vi "niDTS BT Tx Test Example.vi"() -> ()   [LabVIEW 2014]
uses:
  Tx Test/Includes/niDTS BT Tx Test INC IBE Results.ctl
  Tx Test/Includes/niDTS BT Tx Test INC Character Results.ctl
  Tx Test/Includes/niDTS BT Tx Test INC CFO Resutls.ctl
  Tx Test/Includes/niDTS BT Tx Test INC TXP Results.ctl
  Tx Test/Includes/niDTS BT Tx Test INC OBW Results.ctl
  BDR Tx Test/Includes/niDTS BT BDR Tx Test INC Results.ctl
  CommLib/Includes/niDTS Comm INC CLI Login.ctl
  EDR Tx Test/Includes/niDTS BT EDR Tx Test INC Results.ctl
  Tx Test/Includes/niDTS BT Tx Test INC DEVM Results.ctl
  Tx Test/Includes/niDTS BT Tx Test INC CF Stability Results.ctl
  LE Tx Test/Includes/niDTS BT LE Tx Test INC Results.ctl
  LE Tx Test/Includes/niDTS BT LE Tx Test INC Parameters.ctl
  Tx Test/Includes/niDTS BT Tx Test INC BD Payload Data.ctl
  Tx Test/Includes/niDTS BT Tx Test INC Modulation Characteristics.ctl
  Includes/niDTS BT INC TXP Measurement Parameters.ctl
  LE Tx Test/Includes/niDTS BT INC LE IBE Measurement Parameters.ctl
  Includes/niDTS BT DUT INC Trigger.ctl
  EDR Tx Test/Includes/niDTS BT EDR Tx Test INC Parameters.ctl
  EDR Tx Test/Includes/niDTS BT INC EDR Packet Type.ctl
  EDR Tx Test/Includes/niDTS BT INC EDR Data Rate.ctl
  EDR Tx Test/Includes/niDTS BT INC EDR Burst Sync.ctl
  EDR Tx Test/Includes/niDTS BT INC EDR ModAcc Measurement Parameters.ctl
  EDR Tx Test/Includes/niDTS BT INC EDR IBE Measurement Parameters.ctl
  BDR Tx Test/Includes/niDTS BT BDR Tx Test INC Parameters.ctl
  BDR Tx Test/Includes/niDTS BT INC BDR Packet Type.ctl
  Includes/niDTS BT INC OBW Measurement Parameters.ctl
  BDR Tx Test/Includes/niDTS BT INC BDR ACP Measurement Parameters.ctl
  Framework/Logger/Includes/niDTS Logger INC File Parameters.ctl
  TestStand/Station/Objects/SystemDutHandle/niDTS SystemDutHandle.lvclass
  Framework/niDTS Framework.lvlib
  niDTS BT.lvlib
  TestStand/niDTS TestStand.lvlib
  Plugins/niBCM4350 BT/niBCM4350 BT.lvlib
  Plugins/niLEDTM BT/niLEDTM BT.lvlib
  Plugins/niWTM Loopback/niWTM Loopback.lvlib
  Framework/Logger/Listener/Viewer/niDTS Logger Listener Viewer.lvclass
  CommLib/niDTS CommLib.lvlib
panel:
  in  "Keep Log Open":bool
  in  "ResultsIndex":u8=1
  in  "Tab Control":enum32{"BDR", "EDR", "LE TP"}(tab)
  out "BDR Results":T6={"ACP Results"={"Measurement Status"=TRUE, "Reference Channel Power (dBm)"=-9.745, "Upper Channel Power (dBm)"=-37.144, "Lower Channel Power (dBm)"=-37.251, "Total Channel Powers (dBm)"=[-83.632, -78.931, -37.144, -9.745, -37.251, -79.301, -83.479]}, "DF1/DF2"={"Average df1Avg (Hz)"=161011.015625, "Max df1Max (Hz)"=161733.942382812, "Min df1Max (Hz)"=160248.126464844, "Measurement Status df1"=TRUE, "Average  df2Avg/Average df1Avg"=nan, "Average df2Avg (Hz)"=nan, "Max df2Max (Hz)"=nan, "Min df2Max (Hz)"=nan, "Measurement Status df2"=FALSE}, "CFO"={"Max ICFT (Hz)"=548.11181640625, "Max Carrier Drift (Hz)"=-686.029418945312, "Max Carrier Drift/50us (Hz)"=173.238983154297, "LE MaxPayloadBlockFreqOffset (Hz)"=nan, "LE MaxCarrierDrift/55us (Hz)"=nan}, "TXP Resutls"={"Average Burst Power (dBm)"=-9.843, "Peak Burst Power (dBm)"=-9.8, "EdrRelativePower (dB)"=-0.01}, "OBW Resutls"={"OBW (Hz)"=908872.719017752, "Start Frequency (Hz)"=-438547.728652488, "Stop Frequency (Hz)"=470324.990365264}} {"OBW Resutls"."Stop Frequency (Hz)" format="%#_4p"; "OBW Resutls"."Start Frequency (Hz)" format="%#_4p"}
  out "USL":T7={"ACP Results"={"Measurement Status"=FALSE, "Reference Channel Power (dBm)"=23.0, "Upper Channel Power (dBm)"=-20.0, "Lower Channel Power (dBm)"=-20.0, "Total Channel Powers (dBm)"=[]}, "DF1/DF2"={"Average df1Avg (Hz)"=175000.0, "Max df1Max (Hz)"=inf, "Min df1Max (Hz)"=inf, "Measurement Status df1"=FALSE, "Average  df2Avg/Average df1Avg"=inf, "Average df2Avg (Hz)"=175000.0, "Max df2Max (Hz)"=inf, "Min df2Max (Hz)"=inf, "Measurement Status df2"=FALSE}, "CFO"={"Max ICFT (Hz)"=75000.0, "Max Carrier Drift (Hz)"=40000.0, "Max Carrier Drift/50us (Hz)"=20000.0, "LE MaxPayloadBlockFreqOffset (Hz)"=nan, "LE MaxCarrierDrift/55us (Hz)"=nan}, "TXP Resutls"={"Average Burst Power (dBm)"=20.0, "Peak Burst Power (dBm)"=23.0, "EdrRelativePower (dB)"=inf}, "OBW Resutls"={"OBW (Hz)"=1500000.0, "Start Frequency (Hz)"=0.0, "Stop Frequency (Hz)"=750000.0}} {"OBW Resutls"."Stop Frequency (Hz)" format="%#_4p"; "OBW Resutls"."Start Frequency (Hz)" format="%#_4p"}
  out "LSL":T7={"ACP Results"={"Measurement Status"=FALSE, "Reference Channel Power (dBm)"=-inf, "Upper Channel Power (dBm)"=-inf, "Lower Channel Power (dBm)"=-inf, "Total Channel Powers (dBm)"=[]}, "DF1/DF2"={"Average df1Avg (Hz)"=140000.0, "Max df1Max (Hz)"=-inf, "Min df1Max (Hz)"=-inf, "Measurement Status df1"=FALSE, "Average  df2Avg/Average df1Avg"=-inf, "Average df2Avg (Hz)"=-inf, "Max df2Max (Hz)"=115000.0, "Min df2Max (Hz)"=0.0, "Measurement Status df2"=FALSE}, "CFO"={"Max ICFT (Hz)"=-75000.0, "Max Carrier Drift (Hz)"=-40000.0, "Max Carrier Drift/50us (Hz)"=-20000.0, "LE MaxPayloadBlockFreqOffset (Hz)"=nan, "LE MaxCarrierDrift/55us (Hz)"=nan}, "TXP Resutls"={"Average Burst Power (dBm)"=-inf, "Peak Burst Power (dBm)"=-inf, "EdrRelativePower (dB)"=-inf}, "OBW Resutls"={"OBW (Hz)"=0.0, "Start Frequency (Hz)"=-750000.0, "Stop Frequency (Hz)"=0.0}} {"OBW Resutls"."Stop Frequency (Hz)" format="%#_4p"; "OBW Resutls"."Start Frequency (Hz)" format="%#_4p"}
  out "x > y?":T8={"ACP Results"={"Measurement Status"=TRUE, "Reference Channel Power dBm"=TRUE, "Upper Channel Power dBm"=TRUE, "Lower Channel Power dBm"=TRUE, "Total Channel Powers dBm"=[]}, "DF1/DF2"={"Average df1Avg"=TRUE, "Max df1Max"=TRUE, "Min df1Max"=TRUE, "Measurement Status df1"=TRUE, "Average  df2Avg/Average df1Avg"=FALSE, "Average df2Avg"=FALSE, "Max df2Max"=FALSE, "Min df2Max 2"=FALSE, "Measurement Status df2"=FALSE}, "CFO"={"Max ICFT Hz"=TRUE, "Max Carrier Drift Hz"=TRUE, "Max Carrier Drift/50us Hz"=TRUE, "LE Max Block Freq Offset, Hz"=FALSE, "LE Max Carrier Drift/55us Hz"=FALSE}, "TXP Resutls"={"Average Burst Power"=TRUE, "Peak Burst Power"=TRUE, "EdrRelativePower"=TRUE}, "OBW Resutls"={"OBW"=TRUE, "Start Frequency"=TRUE, "Stop Frequency"=TRUE}}
  out "x < y?":T8={"ACP Results"={"Measurement Status"=FALSE, "Reference Channel Power dBm"=TRUE, "Upper Channel Power dBm"=TRUE, "Lower Channel Power dBm"=TRUE, "Total Channel Powers dBm"=[]}, "DF1/DF2"={"Average df1Avg"=TRUE, "Max df1Max"=TRUE, "Min df1Max"=TRUE, "Measurement Status df1"=FALSE, "Average  df2Avg/Average df1Avg"=FALSE, "Average df2Avg"=FALSE, "Max df2Max"=FALSE, "Min df2Max 2"=FALSE, "Measurement Status df2"=FALSE}, "CFO"={"Max ICFT Hz"=TRUE, "Max Carrier Drift Hz"=TRUE, "Max Carrier Drift/50us Hz"=TRUE, "LE Max Block Freq Offset, Hz"=FALSE, "LE Max Carrier Drift/55us Hz"=FALSE}, "TXP Resutls"={"Average Burst Power"=TRUE, "Peak Burst Power"=TRUE, "EdrRelativePower"=TRUE}, "OBW Resutls"={"OBW"=TRUE, "Start Frequency"=TRUE, "Stop Frequency"=TRUE}}
  in  "BDR Tx Input Parameters":T9={"Channel"=0, "Dut Tx Power (dBm)"=-10.0, "Auto Level"=FALSE, "External Attenuation (dB)"=0.0, "BDR Packet type"=enum."DH1", "Payload Data"=enum."AUTO", "Burst Sync"=enum."PREamble", "Packet length (bytes)"=-1, "BD ADDRESS"="\u0000\u0000\u0000\u0000\u0000\u0000000000000000", "Modulation Measurement"={"ModAcc Enable"=TRUE, "CFO Enable"=TRUE, "Character Select"=enum."BOTH", "Averages"=1, "Averaging Mode"=enum."RMS", "Measurement Duration (Symbols)"=-1, "Measurement Offset (Symbols)"=0}, "Trace Enable"=FALSE, "OBW Measurement"={"OBW Enable"=TRUE, "OBW Averages"=1, "Averaging Type"=enum."RMS", "Measurement Interval Mode"=enum."AUTO", "Measurement Interval Length (sec)"=0.005}, "TXP Measurement"={"TXP Power Enable"=TRUE, "TXP Averages"=1, "Averaging Type"=enum."RMS"}, "IBE Measurement"={"IBE Enable"=TRUE, "IBE Averages"=1, "Averaging Type"=enum."RMS", "Numbe of Channels"=7, "Channel Mode"=enum."Centered", "Measurement Interval Mode"=enum."AUTO", "Measurement Interval Length (sec)"=0.005}, "Trigger"={"MinQuietTimeDuration (sec)"=0.0001, "TriggerDelay (sec)"=0.0, "TriggerEdge"=enum."RISing", "TriggerSource"=enum."RF0", "TriggerThreshold (dB)"=-20.0, "TriggerTimeout (sec)"=10.0}} {"Trigger"."MinQuietTimeDuration (sec)" format="%#_6p"}
  out "USL EDR":T17={"IBE Results"={"Measurement Status"=FALSE, "Reference Channel Power (dBm)"=23.0, "Upper Channel Power (dBm)"=-20.0, "Lower Channel Power (dBm)"=-20.0, "Total Channel Powers (dBm)"=[]}, "DEVM"={"Average RMS DEVM (%)"=20.0, "Max Peak DEVM (%)"=35.0, "99% DEVM (%)"=30.0}, "CF Stability"={"Average Inital Freq Error (Hz)"=75000.0, "Max Initial Freq Error (Hz)"=75000.0, "Average Block Abs Freq Error (Hz)"=75000.0, "Max Block Abs Freq Error (Hz)"=75000.0, "Average Block Rel Freq Error (Hz)"=10000.0, "MaxBlockRel Freq Error (Hz)"=10000.0}, "TXP Resutls"={"Average Burst Power (dBm)"=23.0, "Peak Burst Power (dBm)"=20.0, "EdrRelativePower (dB)"=4.0}}
  out "EDR Results":T20
  out "LSL EDR":T17={"IBE Results"={"Measurement Status"=FALSE, "Reference Channel Power (dBm)"=-inf, "Upper Channel Power (dBm)"=-inf, "Lower Channel Power (dBm)"=-inf, "Total Channel Powers (dBm)"=[]}, "DEVM"={"Average RMS DEVM (%)"=0.0, "Max Peak DEVM (%)"=0.0, "99% DEVM (%)"=0.0}, "CF Stability"={"Average Inital Freq Error (Hz)"=-75000.0, "Max Initial Freq Error (Hz)"=-75000.0, "Average Block Abs Freq Error (Hz)"=-75000.0, "Max Block Abs Freq Error (Hz)"=-75000.0, "Average Block Rel Freq Error (Hz)"=-10000.0, "MaxBlockRel Freq Error (Hz)"=-10000.0}, "TXP Resutls"={"Average Burst Power (dBm)"=-inf, "Peak Burst Power (dBm)"=-inf, "EdrRelativePower (dB)"=-1.0}}
  out "EDR":T21
  out "EDR":T21
  in  "EDR Tx Input Parameters":T22={"Channel"=0, "Dut Tx Power  (dBm)"=-10.0, "Auto Level"=FALSE, "External Attenuation (dB)"=0.0, "EDR Packet type"=enum."DH1", "Data Rate"=2, "Payload Data"=enum."PN9", "Burst Sync"=enum."PREamble", "Packet Length, bytes"=-1, "BD ADDRESS"="\u0000\u0000\u0000\u0000\u0000\u0000000000000000", "Trace Enable"=FALSE, "EDR ModAcc Measurement"={"DEVM Enable"=TRUE, "Averages"=1, "Averaging Mode"=enum."RMS", "Measurement Duration (bytes)"=-1, "Measurement Offset (bytes)"=0}, "TXP Measurement"={"TXP Power Enable"=TRUE, "TXP Averages"=1, "Averaging Type"=enum."RMS"}, "IBE  Measurement"={"IBE Enable"=TRUE, "IBE Averages"=1, "Averaging Type"=enum."RMS", "Numbe of Channels"=7, "Channel Mode"=enum."Centered", "Measurement Interval Mode"=enum."AUTO", "Measurement Interval Length (sec)"=0.005}, "Trigger"={"MinQuietTimeDuration (sec)"=0.0001, "TriggerDelay (sec)"=0.0, "TriggerEdge"=enum."RISing", "TriggerSource"=enum."RF0", "TriggerThreshold (dB)"=-20.0, "TriggerTimeout (sec)"=10.0}} {"Trigger"."MinQuietTimeDuration (sec)" format="%#_6p"; "Data Rate" min=2 max=3 step=1}
  out "LE USL":T28={"LE IBE Results"={"Measurement Status"=FALSE, "Reference Channel Power (dBm)"=13.0, "Upper Channel Power (dBm)"=-20.0, "Lower Channel Power (dBm)"=-20.0, "Total Channel Powers (dBm)"=[]}, "DF1/DF2"={"Average df1Avg (Hz)"=nan, "Max df1Max (Hz)"=nan, "Min df1Max (Hz)"=nan, "Measurement Status df1"=FALSE, "Average  df2Avg/Average df1Avg"=inf, "Average df2Avg (Hz)"=nan, "Max df2Max (Hz)"=nan, "Min df2Max (Hz)"=nan, "Measurement Status df2"=FALSE}, "CFO"={"Max ICFT (Hz)"=inf, "Max Carrier Drift (Hz)"=inf, "Max Carrier Drift/50us (Hz)"=inf, "LE MaxPayloadBlockFreqOffset (Hz)"=0.0, "LE MaxCarrierDrift/55us (Hz)"=0.0}, "TXP Resutls"={"Average Burst Power (dBm)"=23.0, "Peak Burst Power (dBm)"=20.0, "EdrRelativePower (dB)"=inf}}
  out "LE LSL":T28={"LE IBE Results"={"Measurement Status"=FALSE, "Reference Channel Power (dBm)"=-inf, "Upper Channel Power (dBm)"=-inf, "Lower Channel Power (dBm)"=-inf, "Total Channel Powers (dBm)"=[]}, "DF1/DF2"={"Average df1Avg (Hz)"=nan, "Max df1Max (Hz)"=nan, "Min df1Max (Hz)"=nan, "Measurement Status df1"=FALSE, "Average  df2Avg/Average df1Avg"=-inf, "Average df2Avg (Hz)"=nan, "Max df2Max (Hz)"=nan, "Min df2Max (Hz)"=nan, "Measurement Status df2"=FALSE}, "CFO"={"Max ICFT (Hz)"=-inf, "Max Carrier Drift (Hz)"=-inf, "Max Carrier Drift/50us (Hz)"=-inf, "LE MaxPayloadBlockFreqOffset (Hz)"=0.0, "LE MaxCarrierDrift/55us (Hz)"=0.0}, "TXP Resutls"={"Average Burst Power (dBm)"=-inf, "Peak Burst Power (dBm)"=-inf, "EdrRelativePower (dB)"=-inf}}
  out "LE Results":T28
  out "x > y?":T29
  out "x < y?":T29
  in  "LE Tx Input Parameters":T30={"Channel"=0, "Dut Tx Power (dBm)"=-10.0, "Auto Level"=FALSE, "External Attenuation (dB)"=0.0, "Payload Data"=enum."AUTO", "Burst Sync"=enum."PREamble", "Packet Length (bytes)"=-1, "Modulation Measurement"={"ModAcc Enable"=TRUE, "CFO Enable"=TRUE, "Character Select"=enum."BOTH", "Averages"=1, "Averaging Mode"=enum."RMS", "Measurement Duration (bytes)"=-1, "Measurement Offset (bytes)"=0}, "TXP Measurement"={"TXP Power Enable"=TRUE, "TXP Averages"=1, "Averaging Type"=enum."RMS"}, "LE IBE Measurement"={"LE IBE Enable"=TRUE, "LE IBE Averages"=1, "Averaging Type"=enum."RMS", "Numbe of Channels"=7, "Channel Mode"=enum."Centered", "Measurement Interval Mode"=enum."AUTO", "Measurement Interval Length (sec)"=0.005}, "Trace Enable"=FALSE, "Trigger"={"MinQuietTimeDuration (sec)"=0.0001, "TriggerDelay (sec)"=0.0, "TriggerEdge"=enum."RISing", "TriggerSource"=enum."RF0", "TriggerThreshold (dB)"=-30.0, "TriggerTimeout (sec)"=10.0}} {"Trigger"."MinQuietTimeDuration (sec)" format="%#_6p"}
  in  "General Parameters":T33={"Port Parameters Serial"={"baud rate "=115200, "data bits"=8, "Enable Termination Char"=TRUE, "flow control"=0, "parity"=enum."None", "timeout (ms) "=5000, "stop bits"=10, "termination char"=10}, "CLI Login"={"Do Login"=FALSE, "Login Prompt"="", "Password"="", "User Name"=""}}
  in  "Socket Index":i32
  in  "System Configuration Path":path=path "C:/Users/Public/Documents/National Instruments/WTM 1.0/System Configurations"
  in  "DUT Plugin":enum32{"LE DTM", "BCM4350", "Loopback"}(tab)=enum."Loopback"
  in  "Interfaces LE DTM":enum32{"Serial", "Other"}(tab)
  in  "Sockets":T34(array[cluster])=[{"BT"={"Serial Resource"="COM5"}}]
  in  "Interfaces BCM4350":enum32{"Serial", "Other"}(tab)
  in  "Sockets":T34(array[cluster])=[{"BT"={"Serial Resource"="COM5"}}]
  in  "Socket Parameters":T35={"Bluetooth"={"VISA Resource"="TCPIP0::InstrumentAddress::inst0::INSTR", "PortNames "=["Port0"]}}
  out "error out":errorcluster
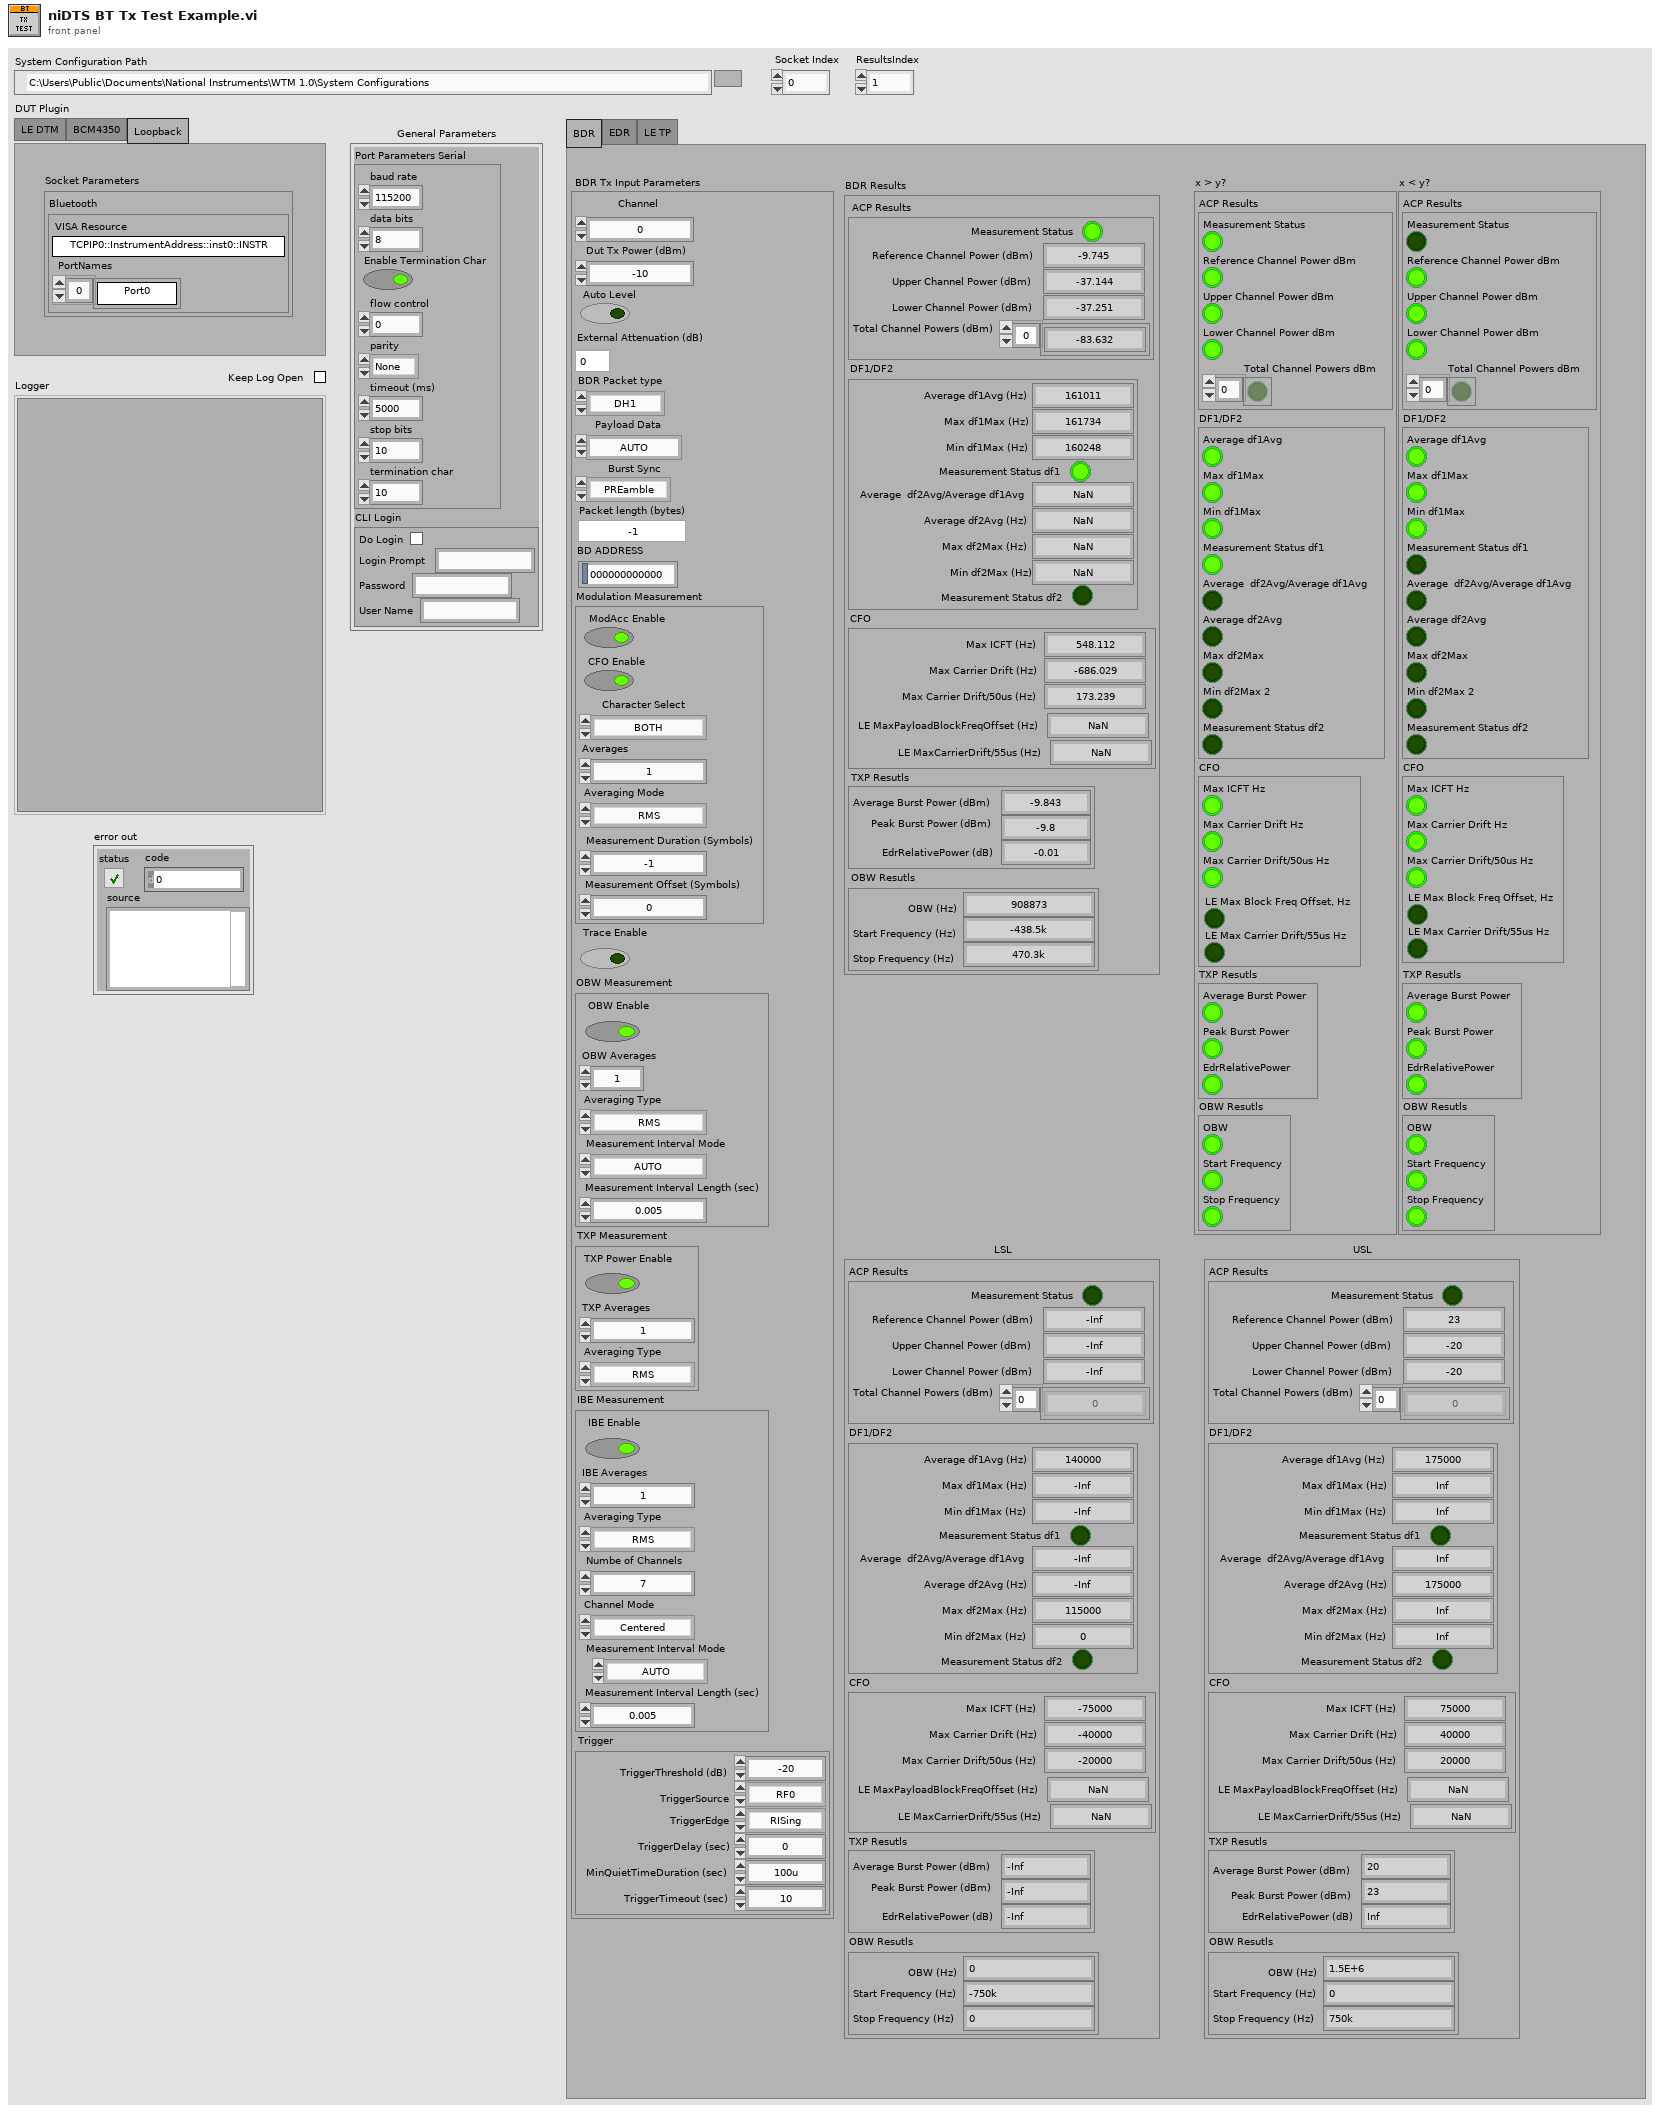
[diagram p1: front panel]
types:
  T1 = typedef "niDTS BT.lvlib/niDTS BT Tx Test INC IBE Results.ctl" = cluster{"Measurement Status":bool, "Reference Channel Power (dBm)":dbl, "Upper Channel Power (dBm)":dbl, "Lower Channel Power (dBm)":dbl, "Total Channel Powers (dBm)":dbl[]}
  T2 = typedef "niDTS BT.lvlib/niDTS BT Tx Test INC Character Results.ctl" = cluster{"Average df1Avg (Hz)":dbl, "Max df1Max (Hz)":dbl, "Min df1Max (Hz)":dbl, "Measurement Status df1":bool, "Average  df2Avg/Average df1Avg":dbl, "Average df2Avg (Hz)":dbl, "Max df2Max (Hz)":dbl, "Min df2Max (Hz)":dbl, "Measurement Status df2":bool}
  T3 = typedef "niDTS BT.lvlib/niDTS BT Tx Test INC CFO Resutls.ctl" = cluster{"Max ICFT (Hz)":dbl, "Max Carrier Drift (Hz)":dbl, "Max Carrier Drift/50us (Hz)":dbl, "LE MaxPayloadBlockFreqOffset (Hz)":dbl, "LE MaxCarrierDrift/55us (Hz)":dbl}
  T4 = typedef "niDTS BT.lvlib/niDTS BT Tx Test INC TXP Results.ctl" = cluster{"Average Burst Power (dBm)":dbl, "Peak Burst Power (dBm)":dbl, "EdrRelativePower (dB)":dbl}
  T5 = typedef "niDTS BT.lvlib/niDTS BT Tx Test INC OBW Results.ctl" = cluster{"OBW (Hz)":dbl, "Start Frequency (Hz)":dbl, "Stop Frequency (Hz)":dbl}
  T6 = cluster{"ACP Results":T1, "DF1/DF2":T2, "CFO":T3, "TXP Resutls":T4, "OBW Resutls":T5}
  T7 = typedef "niDTS BT.lvlib/niDTS BT BDR Tx Test INC Results.ctl" = cluster{"ACP Results":T1, "DF1/DF2":T2, "CFO":T3, "TXP Resutls":T4, "OBW Resutls":T5}
  T8 = cluster{"ACP Results":cluster{"Measurement Status":bool, "Reference Channel Power dBm":bool, "Upper Channel Power dBm":bool, "Lower Channel Power dBm":bool, "Total Channel Powers dBm":bool[]}, "DF1/DF2":cluster{"Average df1Avg":bool, "Max df1Max":bool, "Min df1Max":bool, "Measurement Status df1":bool, "Average  df2Avg/Average df1Avg":bool, "Average df2Avg":bool, "Max df2Max":bool, "Min df2Max 2":bool, "Measurement Status df2":bool}, "CFO":cluster{"Max ICFT Hz":bool, "Max Carrier Drift Hz":bool, "Max Carrier Drift/50us Hz":bool, "LE Max Block Freq Offset, Hz":bool, "LE Max Carrier Drift/55us Hz":bool}, "TXP Resutls":cluster{"Average Burst Power":bool, "Peak Burst Power":bool, "EdrRelativePower":bool}, "OBW Resutls":cluster{"OBW":bool, "Start Frequency":bool, "Stop Frequency":bool}}
  T9 = typedef "niDTS BT.lvlib/niDTS BT BDR Tx Test INC Parameters.ctl" = cluster{"Channel":i32, "Dut Tx Power (dBm)":dbl, "Auto Level":bool, "External Attenuation (dB)":dbl, "BDR Packet type":T10, "Payload Data":T11, "Burst Sync":enum16{"NONE", "PREamble"}, "Packet length (bytes)":i32, "BD ADDRESS":string, "Modulation Measurement":cluster{"ModAcc Enable":bool, "CFO Enable":bool, "Character Select":T12, "Averages":i32, "Averaging Mode":enum16{"RMS", "LOG", "SCALAR", "MAX", "MIN", "VECTOR"}, "Measurement Duration (Symbols)":i32, "Measurement Offset (Symbols)":i32}, "Trace Enable":bool, "OBW Measurement":T13, "TXP Measurement":T14, "IBE Measurement":T15, "Trigger":T16}
  T10 = typedef "niDTS BT.lvlib/niDTS BT INC BDR Packet Type.ctl" = enum16{"NULL", "POLL", "FHS", "DM1", "DH1", "HV1", "HV2", "HV3", "EV3", "DV", "AUX1", "DM3", "DH3", "EV4", "EV5", "DM5", "DH5"}
  T11 = typedef "niDTS BT.lvlib/niDTS BT Tx Test INC BD Payload Data.ctl" = enum16{"0", "1", "01", "00001111", "PN9", "AUTO"}
  T12 = typedef "niDTS BT.lvlib/niDTS BT Tx Test INC Modulation Characteristics.ctl" = enum16{"DF1", "DF2", "BOTH"}
  T13 = typedef "niDTS BT.lvlib/niDTS BT INC OBW Measurement Parameters.ctl" = cluster{"OBW Enable":bool, "OBW Averages":i32, "Averaging Type":enum16{"RMS", "LOG", "SCALAR", "MAX", "MIN", "VECTOR"}, "Measurement Interval Mode":enum16{"AUTO", "MANUAL"}, "Measurement Interval Length (sec)":dbl}
  T14 = typedef "niDTS BT.lvlib/niDTS BT INC TXP Measurement Parameters.ctl" = cluster{"TXP Power Enable":bool, "TXP Averages":i32, "Averaging Type":enum16{"RMS", "LOG", "SCALAR", "MAX", "MIN"}}
  T15 = typedef "niDTS BT.lvlib/niDTS BT INC BDR ACP Measurement Parameters.ctl" = cluster{"IBE Enable":bool, "IBE Averages":i32, "Averaging Type":enum16{"RMS", "LOG", "SCALAR", "MAX", "MIN", "VECTOR"}, "Numbe of Channels":i32, "Channel Mode":enum16{"InBand", "Centered"}, "Measurement Interval Mode":enum16{"AUTO", "MANUAL"}, "Measurement Interval Length (sec)":dbl}
  T16 = typedef "niDTS BT.lvlib/niDTS BT DUT INC Trigger.ctl" = cluster{"MinQuietTimeDuration (sec)":dbl, "TriggerDelay (sec)":dbl, "TriggerEdge":enum16{"RISing", "FALLing"}, "TriggerSource":enum16{"IMMediate", "RF0", "PFI0", "PFI1", "RTS0", "RTS1", "RTS2", "RTS3", "RTS4", "RTS5", "RTS6", "RTS7", "PXIStar", "SOFT"}, "TriggerThreshold (dB)":dbl, "TriggerTimeout (sec)":dbl}
  T17 = typedef "niDTS BT.lvlib/niDTS BT EDR Tx Test INC Results.ctl" = cluster{"IBE Results":T1, "DEVM":T18, "CF Stability":T19, "TXP Resutls":T4}
  T18 = typedef "niDTS BT.lvlib/niDTS BT Tx Test INC DEVM Results.ctl" = cluster{"Average RMS DEVM (%)":dbl, "Max Peak DEVM (%)":dbl, "99% DEVM (%)":dbl}
  T19 = typedef "niDTS BT.lvlib/niDTS BT Tx Test INC CF Stability Results.ctl" = cluster{"Average Inital Freq Error (Hz)":dbl, "Max Initial Freq Error (Hz)":dbl, "Average Block Abs Freq Error (Hz)":dbl, "Max Block Abs Freq Error (Hz)":dbl, "Average Block Rel Freq Error (Hz)":dbl, "MaxBlockRel Freq Error (Hz)":dbl}
  T20 = cluster{"IBE Results":T1, "DEVM":T18, "CF Stability":T19, "TXP Resutls":T4}
  T21 = cluster{"IBE Results":cluster{"Measurement Status":bool, "Reference Channel Power dBm":bool, "Upper Channel Power dBm":bool, "Lower Channel Power dBm":bool, "Total Channel Powers dBm":bool[]}, "DEVM":cluster{"Average RMS DEVM %":bool, "Max Peak DEVM %":bool, "99% DEVM %":bool}, "CF Stability":cluster{"Average Inital Freq Error Hz":bool, "Max Initial Freq Error Hz":bool, "Average Block Abs Freq Error Hz":bool, "Max Block Abs Freq Error Hz":bool, "Average Block Rel Freq Error Hz":bool, "MaxBlockRel Freq Error Hz":bool}, "TXP Resutls":cluster{"Average Burst Power":bool, "Peak Burst Power":bool, "EdrRelativePower":bool}}
  T22 = typedef "niDTS BT.lvlib/niDTS BT EDR Tx Test INC Parameters.ctl" = cluster{"Channel":i32, "Dut Tx Power  (dBm)":dbl, "Auto Level":bool, "External Attenuation (dB)":dbl, "EDR Packet type":T23, "Data Rate":T24, "Payload Data":T11, "Burst Sync":T25, "Packet Length, bytes":i32, "BD ADDRESS":string, "Trace Enable":bool, "EDR ModAcc Measurement":T26, "TXP Measurement":T14, "IBE  Measurement":T27, "Trigger":T16}
  T23 = typedef "niDTS BT.lvlib/niDTS BT INC EDR Packet Type.ctl" = enum16{"NULL", "POLL", "FHS", "DM1", "DH1", "HV1", "HV2", "HV3", "EV3", "DV", "AUX1", "DM3", "DH3", "EV4", "EV5", "DM5", "DH5"}
  T24 = typedef "niDTS BT.lvlib/niDTS BT INC EDR Data Rate.ctl" = i32
  T25 = typedef "niDTS BT.lvlib/niDTS BT INC EDR Burst Sync.ctl" = enum16{"NONE", "PREamble"}
  T26 = typedef "niDTS BT.lvlib/niDTS BT INC EDR ModAcc Measurement Parameters.ctl" = cluster{"DEVM Enable":bool, "Averages":i32, "Averaging Mode":enum16{"RMS", "LOG", "SCALAR", "MAX", "MIN", "VECTOR"}, "Measurement Duration (bytes)":i32, "Measurement Offset (bytes)":i32}
  T27 = typedef "niDTS BT.lvlib/niDTS BT INC EDR IBE Measurement Parameters.ctl" = cluster{"IBE Enable":bool, "IBE Averages":i32, "Averaging Type":enum16{"RMS", "LOG", "SCALAR", "MAX", "MIN", "VECTOR"}, "Numbe of Channels":i32, "Channel Mode":enum16{"InBand", "Centered"}, "Measurement Interval Mode":enum16{"AUTO", "MANUAL"}, "Measurement Interval Length (sec)":dbl}
  T28 = typedef "niDTS BT.lvlib/niDTS BT LE Tx Test INC Results.ctl" = cluster{"LE IBE Results":T1, "DF1/DF2":T2, "CFO":T3, "TXP Resutls":T4}
  T29 = cluster{"LE IBE Results":cluster{"Measurement Status":bool, "Reference Channel Power dBm":bool, "Upper Channel Power dBm":bool, "Lower Channel Power dBm":bool, "Total Channel Powers dBm":bool[]}, "DF1/DF2":cluster{"Average df1Avg":bool, "Max df1Max":bool, "Min df1Max":bool, "Measurement Status df1":bool, "Average  df2Avg/Average df1Avg":bool, "Average df2Avg":bool, "Max df2Max":bool, "Min df2Max 2":bool, "Measurement Status df2":bool}, "CFO":cluster{"Max ICFT Hz":bool, "Max Carrier Drift Hz":bool, "Max Carrier Drift/50us Hz":bool, "LE Max Block Freq Offset, Hz":bool, "LE Max Carrier Drift/55us Hz":bool}, "TXP Resutls":cluster{"Average Burst Power":bool, "Peak Burst Power":bool, "EdrRelativePower":bool}}
  T30 = typedef "niDTS BT.lvlib/niDTS BT LE Tx Test INC Parameters.ctl" = cluster{"Channel":i32, "Dut Tx Power (dBm)":dbl, "Auto Level":bool, "External Attenuation (dB)":dbl, "Payload Data":T11, "Burst Sync":enum16{"NONE", "PREamble"}, "Packet Length (bytes)":i32, "Modulation Measurement":cluster{"ModAcc Enable":bool, "CFO Enable":bool, "Character Select":T12, "Averages":i32, "Averaging Mode":enum16{"RMS", "LOG", "SCALAR", "MAX", "MIN", "VECTOR"}, "Measurement Duration (bytes)":i32, "Measurement Offset (bytes)":i32}, "TXP Measurement":T14, "LE IBE Measurement":T31, "Trace Enable":bool, "Trigger":T16}
  T31 = typedef "niDTS BT.lvlib/niDTS BT INC LE IBE Measurement Parameters.ctl" = cluster{"LE IBE Enable":bool, "LE IBE Averages":i32, "Averaging Type":enum16{"RMS", "LOG", "SCALAR", "MAX", "MIN", "VECTOR"}, "Numbe of Channels":i32, "Channel Mode":enum16{"InBand", "Centered"}, "Measurement Interval Mode":enum16{"AUTO", "MANUAL"}, "Measurement Interval Length (sec)":dbl}
  T32 = typedef "niDTS CommLib.lvlib/niDTS Comm INC CLI Login.ctl" = cluster{"Do Login":bool, "Login Prompt":string, "Password":string, "User Name":string}
  T33 = cluster{"Port Parameters Serial":cluster{"baud rate ":u32, "data bits":u16, "Enable Termination Char":bool, "flow control":u16, "parity":enum16{"None", "Odd", "Even", "Mark", "Space"}, "timeout (ms) ":u32, "stop bits":u16, "termination char":u8}, "CLI Login":T32}
  T34 = cluster{"BT":cluster{"Serial Resource":refnum<visa-resource-name>}}[]
  T35 = cluster{"Bluetooth":cluster{"VISA Resource":string, "PortNames ":string[]}}
  T36 = typedef "niDTS Framework.lvlib/niDTS Logger INC File Parameters.ctl" = cluster{"File Size (Bytes)":u32, "New File Per Day":bool, "File Location":path, "Base File Name":string}
  T37 = typedef "niDTS Framework.lvlib/niDTS Logger INC Handle.ctl" = refnum<data-value>
  T38 = cluster{"WLAN":cluster{"VISA Resource":string, "PortNames ":string[]}, "Bluetooth":cluster{"VISA Resource":string, "PortNames ":string[]}, "GNSS":cluster{"VISA Resource":string, "PortNames ":string[]}}
  T39 = cluster{"BT":cluster{"Serial Resource":refnum<visa-resource-name>}}
  T40 = cluster{"VISA Resource":string, "PortNames ":string[]}
  T41 = typedef "niDTS TestStand.lvlib/niDTS SystemDutHandle.lvclass/niDTS SystemDutHandle INC SystemDutHandles.ctl" = refnum<class "niDTS SystemDutHandle.lvclass">[]
  T42 = typedef "niDTS Framework.lvlib/niDTS Dut INC Handle.ctl" = refnum<data-value>
  T43 = typedef "niDTS BT.lvlib/niDTS BT Tx Test INC Handle.ctl" = refnum<data-value>
  T44 = cluster{"ACP Results":cluster{"Measurement Status":bool, "Reference Channel Power (dBm)":bool, "Upper Channel Power (dBm)":bool, "Lower Channel Power (dBm)":bool, "Total Channel Powers (dBm)":bool[]}, "DF1/DF2":cluster{"Average df1Avg (Hz)":bool, "Max df1Max (Hz)":bool, "Min df1Max (Hz)":bool, "Measurement Status df1":bool, "Average  df2Avg/Average df1Avg":bool, "Average df2Avg (Hz)":bool, "Max df2Max (Hz)":bool, "Min df2Max (Hz)":bool, "Measurement Status df2":bool}, "CFO":cluster{"Max ICFT (Hz)":bool, "Max Carrier Drift (Hz)":bool, "Max Carrier Drift/50us (Hz)":bool, "LE MaxPayloadBlockFreqOffset (Hz)":bool, "LE MaxCarrierDrift/55us (Hz)":bool}, "TXP Resutls":cluster{"Average Burst Power (dBm)":bool, "Peak Burst Power (dBm)":bool, "EdrRelativePower (dB)":bool}, "OBW Resutls":cluster{"OBW (Hz)":bool, "Start Frequency (Hz)":bool, "Stop Frequency (Hz)":bool}}
  T45 = cluster{"IBE Results":cluster{"Measurement Status":bool, "Reference Channel Power (dBm)":bool, "Upper Channel Power (dBm)":bool, "Lower Channel Power (dBm)":bool, "Total Channel Powers (dBm)":bool[]}, "DEVM":cluster{"Average RMS DEVM (%)":bool, "Max Peak DEVM (%)":bool, "99% DEVM (%)":bool}, "CF Stability":cluster{"Average Inital Freq Error (Hz)":bool, "Max Initial Freq Error (Hz)":bool, "Average Block Abs Freq Error (Hz)":bool, "Max Block Abs Freq Error (Hz)":bool, "Average Block Rel Freq Error (Hz)":bool, "MaxBlockRel Freq Error (Hz)":bool}, "TXP Resutls":cluster{"Average Burst Power (dBm)":bool, "Peak Burst Power (dBm)":bool, "EdrRelativePower (dB)":bool}}
  T46 = cluster{"LE IBE Results":cluster{"Measurement Status":bool, "Reference Channel Power (dBm)":bool, "Upper Channel Power (dBm)":bool, "Lower Channel Power (dBm)":bool, "Total Channel Powers (dBm)":bool[]}, "DF1/DF2":cluster{"Average df1Avg (Hz)":bool, "Max df1Max (Hz)":bool, "Min df1Max (Hz)":bool, "Measurement Status df1":bool, "Average  df2Avg/Average df1Avg":bool, "Average df2Avg (Hz)":bool, "Max df2Max (Hz)":bool, "Min df2Max (Hz)":bool, "Measurement Status df2":bool}, "CFO":cluster{"Max ICFT (Hz)":bool, "Max Carrier Drift (Hz)":bool, "Max Carrier Drift/50us (Hz)":bool, "LE MaxPayloadBlockFreqOffset (Hz)":bool, "LE MaxCarrierDrift/55us (Hz)":bool}, "TXP Resutls":cluster{"Average Burst Power (dBm)":bool, "Peak Burst Power (dBm)":bool, "EdrRelativePower (dB)":bool}}
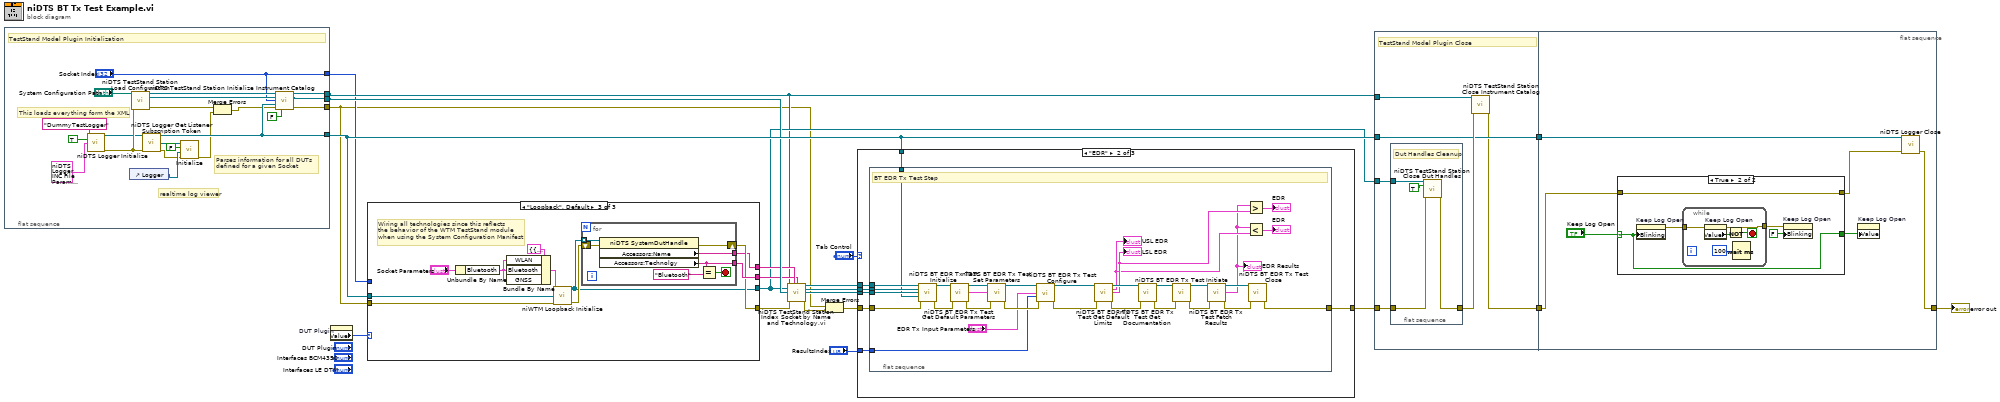
[diagram p0: block diagram]
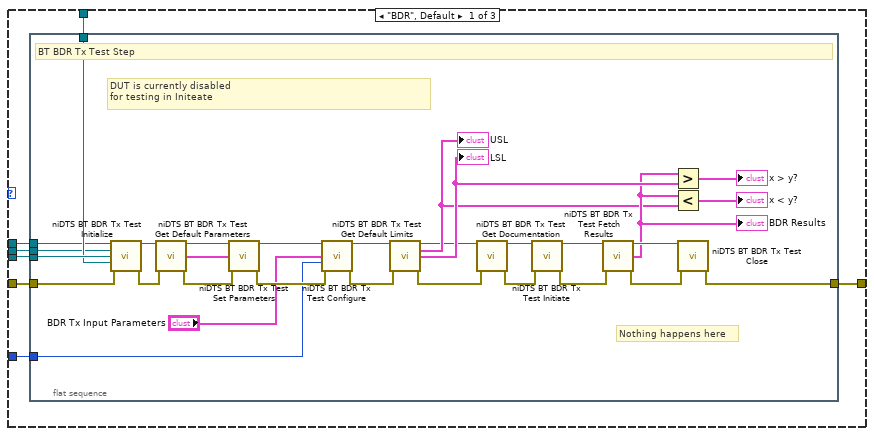
[diagram p2: hidden frame]
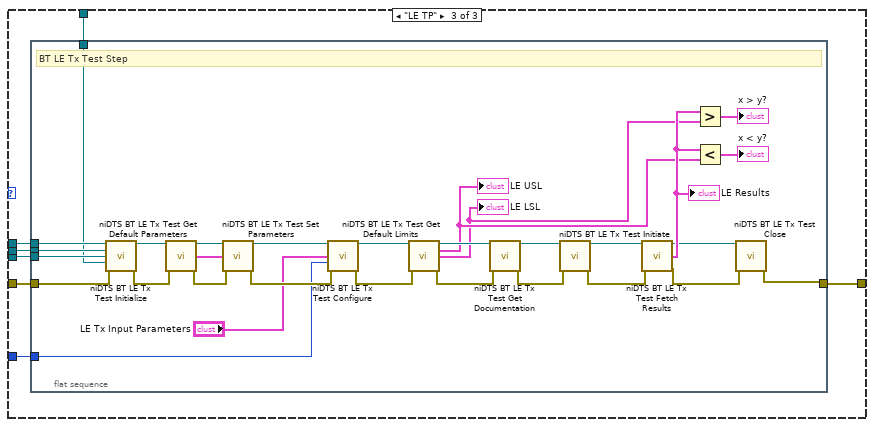
[diagram p3: hidden frame]
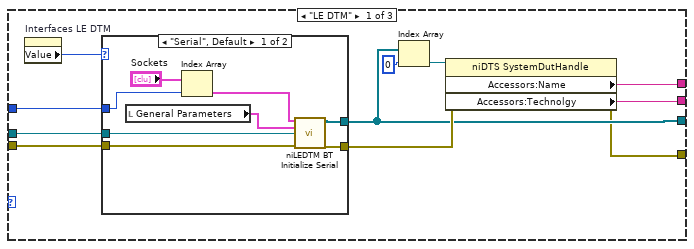
[diagram p4: hidden frame]
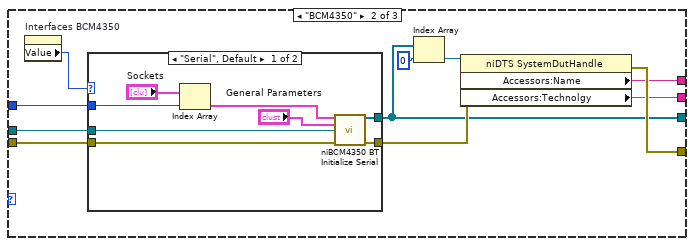
[diagram p6: hidden frame]
diagram:
  n1 = flat-sequence {
    tunnel: [w25] -> w18
    tunnel: [w34] -> w3
    tunnel: [w36] -> w17
    tunnel: [w35] -> w11
    tunnel: ["Socket Index"] -> w8
    frame #0 {
      # "realtime log viewer"
      # "Parses information for all DUTs defined for a given Socket"
      # "This loads everything form the XML"
      # "TestStand Model Plugin Initialization"
      n2 = call "niDTS Logger Initialize.vi"("Session Name ()"="DummyTestLogger", "Log to File"=TRUE, "Logger File Parameters"=T36 {"File Size (Bytes)"=600000, "New File Per Day"=TRUE, "File Location"=path "C:/Logfiles/evm", "Base File Name"=""}) -> ("Logger Handle out"=w26:T37, "error out"=w27:errorcluster)  [unwired: 11 in]
      n3 = control-ref of="Logger"() -> (w31:refnum<vi>)
      n4 = call "niDTS TestStand Station Load Configuration.vi"("System Configuration XML Path"="System Configuration Path", "error in (no error)"=w27) -> ("All System Hardware"=w41:refnum<class "niDTS SystemHardware.lvclass">, "All DUT Definitions"=w39:refnum<class "niDTS SystemDut.lvclass">[], "error out"=w24:errorcluster)  [unwired: 11 in]
      n5 = call "niDTS Logger Get Listener Subscription Token.vi"("Logger Handle in"=w26, "error in (no error)"=w27) -> ("Logger Handle out"=w25:T37, "Listener Subscription Token"=w28:refnum<class "niDTS Logger Listener Subscription Token.lvclass">, "error out"=w29:errorcluster)  [unwired: 11 in]
      n6 = call "Initialize.vi"("error in (no error)"=w29, "SubPanel Reference"=w31, "Open Viewer?"=FALSE, "Listener Subscription Token"=w28) -> ("error out"=w22:errorcluster)  [unwired: 6 in, 1 out]
      n7 = Merge Errors(w24, w22) -> (w23:errorcluster)
      n8 = call "niDTS TestStand Station Initialize Instrument Catalog.vi"("All System Hardware"=w41, "All DUT Definitions"=w39, "Socket Index"="Socket Index", "Logger Handle"=w25, "error in (no error)"=w23, "Simulation Mode (F)"=FALSE) -> ("Socket Instrument Catalog"=w35:refnum<class "niDTS SystemInstrCatalog.lvclass">, "Socket DUT Definitions"=w36:refnum<class "niDTS SystemDut.lvclass">[], "error out"=w34:errorcluster)  [unwired: 7 in]
    }
  }
  n9 = property on="DUT Plugin" class="TabCtl (strict)"() -> ("Value"=w19:enum32{"LE DTM", "BCM4350", "Loopback"})  [unwired: 2 in, 2 out]
  n10 = case shown="\"Loopback\", Default" w19 {
    tunnel: [w43 w68 w91] -> w9
    tunnel: w18 -> [w51 w71 w90]
    tunnel: [w44 w67 w83] -> w12
    tunnel: w3 -> [w50 w72 w89]
    tunnel: [w47 w66 w88] -> w16
    tunnel: [w46 w65 w92] -> w15
    tunnel: w8 -> [w52 w63 _]
    frame "LE DTM" {
      n11 = property on="Interfaces LE DTM" class="TabCtl (strict)"() -> ("Value"=w53:enum32{"Serial", "Other"})  [unwired: 2 in, 2 out]
      n12 = case shown="\"Serial\", Default" w53 {
        tunnel: w52 -> [w60 _]
        tunnel: w51 -> [w58 _]
        tunnel: w50 -> [w57 w62]
        tunnel: [w56 w62] -> w45
        tunnel: [w54 _] -> w44
        frame "Serial", Default {
          n13 = local read "General Parameters"() -> (w59:T33)
          n14 = Index Array(array="Sockets", index=w60) -> (element=w55:T39)
          n15 = call "niLEDTM BT Initialize Serial.vi"("Socket Parameters"=w55, "General Parameters"=w59, "Logger"=w58, "error in (no error)"=w57) -> ("DUT Technology Handles"=w54:refnum<class "niDTS SystemDutHandle.lvclass">[], "Error"=w56:errorcluster)  [unwired: 10 in]
        }
        frame "Other" {
          # "Future Implementation"
        }
      }
      n16 = Index Array(array=w44, index=0) -> (element=w49:refnum<class "niDTS SystemDutHandle.lvclass">)
      n17 = property class="niDTS SystemDutHandle"(reference=w49, error in=w45) -> (error out=w43:errorcluster, "Accessors:Name"=w47:string, "Accessors:Technolgy"=w46:string)  [unwired: 1 out]
    }
    frame "BCM4350" {
      n18 = property on="Interfaces BCM4350" class="TabCtl (strict)"() -> ("Value"=w73:enum32{"Serial", "Other"})  [unwired: 2 in, 2 out]
      n19 = case shown="\"Serial\", Default" w73 {
        tunnel: [w81 _] -> w67
        tunnel: [w80 w82] -> w69
        tunnel: w72 -> [w79 w82]
        tunnel: w71 -> [w78 _]
        tunnel: w63 -> [w75 _]
        frame "Serial", Default {
          n20 = Index Array(array="Sockets", index=w75) -> (element=w74:T39)
          n21 = call "niBCM4350 BT Initialize Serial.vi"("Socket Parameters"=w74, "General Parameters"="General Parameters", "Logger"=w78, "error in (no error)"=w79) -> ("DUT Technology Handles"=w81:refnum<class "niDTS SystemDutHandle.lvclass">[], "Error"=w80:errorcluster)  [unwired: 10 in]
        }
        frame "Other" {
          # "Future Implementation"
        }
      }
      n22 = Index Array(array=w67, index=0) -> (element=w70:refnum<class "niDTS SystemDutHandle.lvclass">)
      n23 = property class="niDTS SystemDutHandle"(reference=w70, error in=w69) -> (error out=w68:errorcluster, "Accessors:Name"=w66:string, "Accessors:Technolgy"=w65:string)  [unwired: 1 out]
    }
    frame "Loopback", Default {
      # "Wiring all technologies since this reflects \nthe behavior of the WTM TestStand module \nwhen using the System Configuration Manifest"
      n24 = Unbundle By Name("Socket Parameters") -> ("Bluetooth"=w84:T40)
      n25 = Bundle By Name(cluster=T38 {"WLAN"={"VISA Resource"="TCPIP0::InstrumentAddress::inst0::INSTR", "PortNames "=["Port0"]}, "Bluetooth"={"VISA Resource"="TCPIP0::InstrumentAddress::inst0::INSTR", "PortNames "=["Port0"]}, "GNSS"={"VISA Resource"="TCPIP0::InstrumentAddress::inst0::INSTR", "PortNames "=["Port0"]}} ("Socket Parameters"), "WLAN"=w84, "Bluetooth"=w84, "GNSS"=w84) -> (w86:T38)
      n26 = call "niWTM Loopback Initialize.vi"("Socket Parameters"=w86, "Logger"=w90, "error in (no error)"=w89) -> ("Dut Technology Handles"=w83:T41, "error out"=w93:errorcluster)  [unwired: 11 in]
      n27 = for {
        tunnel: [w95] -> w92
        tunnel: [w98] -> w88
        shift-right: [w99] -> w91
        shift-left: w93 -> [w100]
        tunnel: w83 -> [w97] mode=indexing
        stop <- w94 stop-if-true
        n28 = property class="niDTS SystemDutHandle"(reference=w97, error in=w100) -> (error out=w99:errorcluster, "Accessors:Name"=w98:string, "Accessors:Technolgy"=w95:string)  [unwired: 1 out]
        n29 = Equal?(x=w95, y="Bluetooth") -> (x = y?=w94:bool)
      }
    }
  }
  n30 = call "niDTS TestStand Station Index Socket by Name and Technology,vi.vi"("niDTS SystemInstrCatalog in"=w11, "Name"=w16, "Technology"=w15, "System Dut Handles"=w12, "Socket DUT Definitions"=w17, "error in (no error)"=w9) -> ("Dut Handle"=w10:T42, "SystemTechnologyCatalog"=w13:refnum<class "niDTS SystemTechnologyCatalog.lvclass">, "Specific Socket/Tech DUT Definition"=w14:refnum<class "niDTS SystemDut.lvclass">, "error out"=w7:errorcluster)  [unwired: 6 in]
  n31 = Merge Errors(w3, w7) -> (w6:errorcluster)
  n32 = case shown="\"EDR\"" "Tab Control" {
    tunnel: [w107 w143 w180] -> w21
    tunnel: w18 -> [w102 w139 w176]
    tunnel: w6 -> [w106 w144 w181]
    tunnel: w14 -> [w105 w141 w178]
    tunnel: w13 -> [w104 w142 w179]
    tunnel: w10 -> [w103 w140 w177]
    tunnel: "ResultsIndex" -> [w101 w138 w175]
    frame "BDR", Default {
      n33 = flat-sequence {
        tunnel: w102 -> [w129]
        tunnel: [w135] -> w107
        tunnel: w106 -> [w130]
        tunnel: w105 -> [w131]
        tunnel: w104 -> [w128]
        tunnel: w103 -> [w127]
        tunnel: w101 -> [w116]
        frame #0 {
          # "DUT is currently disabled\nfor testing in Initeate"
          # "Nothing happens here"
          # "BT BDR Tx Test Step"
          n34 = call "niDTS BT BDR Tx Test  Initialize.vi"("Dut Reference"=w127, "SystemTechnologyCatalog"=w128, "SystemDut"=w131, "Logger Reference"=w129, "error in (no error)"=w130) -> ("Dummy Test Handle out"=w124:T43, "error out"=w123:errorcluster)  [unwired: 8 in, 1 out]
          n35 = call "niDTS BT BDR Tx Test Get Default Parameters.vi"("Dummy Test Handle In"=w124, "error in (no error)"=w123) -> ("Dummy Test Handle Out"=w115:T43, "BDR Tx Parameters"=w113:T9, "error out"=w114:errorcluster)  [unwired: 11 in]
          n36 = call "niDTS BT BDR Tx Test Set Parameters.vi"("Dummy Test Handle In"=w115, "BT BDR Parameters"=w113, "error in (no error)"=w114) -> ("Dummy Test Handle Out"=w126:T43, "error out"=w125:errorcluster)  [unwired: 11 in]
          n37 = call "niDTS BT BDR Tx Test Configure.vi"("Dummy Test Handle In"=w126, "BT BDR Parameters"="BDR Tx Input Parameters", "ResultsIndex"=w116, "error in (no error)"=w125) -> ("Dummy Test Handle Out"=w133:T43, "error out"=w132:errorcluster)  [unwired: 10 in]
          n38 = call "niDTS BT BDR Tx Test Get Default Limits.vi"("Dummy Test Handle In"=w133, "error in (no error)"=w132) -> ("Dummy Test Handle Out"=w112:T43, "USL"=w120:T7, "LSL"=w122:T7, "error out"=w110:errorcluster)  [unwired: 10 in]
          "USL" <- w120
          "LSL" <- w122
          n39 = call "niDTS BT BDR Tx Test Get Documentation.vi"("Dummy Test Handle In"=w112, "error in (no error)"=w110) -> ("Dummy Test Handle Out"=w111:T43, "error out"=w109:errorcluster)  [unwired: 11 in, 1 out]
          n40 = call "niDTS BT BDR Tx Test Initiate.vi"("Dummy Test Handle In"=w111, "error in (no error)"=w109) -> ("Dummy Test Handle Out"=w134:T43, "error out"=w117:errorcluster)  [unwired: 12 in]
          n41 = call "niDTS BT BDR Tx Test Fetch Results.vi"("Dummy Test Handle in"=w134, "error in (no error)"=w117) -> ("Dummy Test Handle out"=w137:T43, "Resutls"=w121:T7, "error out"=w136:errorcluster)  [unwired: 11 in]
          "BDR Results" <- w121
          n42 = Greater?(x=w121, y=w122) -> (0:→"x > y?":T44)
          n43 = Less?(x=w121, y=w120) -> (x < y?=→"x < y?":T44)
          n44 = call "niDTS BT BDR Tx Test Close.vi"("Dummy Test Handle out"=w137, "error in (no error)"=w136) -> ("error out"=w135:errorcluster)  [unwired: 13 in]
        }
      }
    }
    frame "EDR" {
      n45 = flat-sequence {
        tunnel: w144 -> [w174]
        tunnel: [w148] -> w143
        tunnel: w142 -> [w164]
        tunnel: w141 -> [w163]
        tunnel: w140 -> [w162]
        tunnel: w139 -> [w161]
        tunnel: w138 -> [w154]
        frame #0 {
          # "BT EDR Tx Test Step"
          n46 = call "niDTS BT EDR Tx Test  Initialize.vi"("Dut Reference"=w162, "SystemTechnologyCatalog"=w164, "SystemDut"=w163, "Logger Reference"=w161, "error in (no error)"=w174) -> ("Dummy Test Handle out"=w169:T43, "error out"=w173:errorcluster)  [unwired: 8 in, 1 out]
          n47 = call "niDTS BT EDR Tx Test Get Default Parameters.vi"("Dummy Test Handle In"=w169, "error in (no error)"=w173) -> ("Dummy Test Handle Out"=w160:T43, "output cluster"=w146:T22, "error out"=w159:errorcluster)  [unwired: 11 in]
          n48 = call "niDTS BT EDR Tx Test Set Parameters.vi"("Dummy Test Handle In"=w160, "EDR Tx Input Parameters"=w146, "error in (no error)"=w159) -> ("Dummy Test Handle Out"=w158:T43, "error out"=w157:errorcluster)  [unwired: 11 in]
          n49 = call "niDTS BT EDR Tx Test Configure.vi"("Dummy Test Handle In"=w158, "EDR Tx Input Parameters"="EDR Tx Input Parameters", "ResultsIndex"=w154, "error in (no error)"=w157) -> ("Dummy Test Handle Out"=w156:T43, "error out"=w155:errorcluster)  [unwired: 10 in]
          n50 = call "niDTS BT EDR Tx Test Get Default Limits.vi"("Dummy Test Handle In"=w156, "error in (no error)"=w155) -> ("Dummy Test Handle Out"=w168:T43, "USL"=w152:T17, "LSL"=w153:T17, "error out"=w172:errorcluster)  [unwired: 10 in]
          "USL EDR" <- w152
          "LSL EDR" <- w153
          n51 = call "niDTS BT EDR Tx Test Get Documentation.vi"("Dummy Test Handle In"=w168, "error in (no error)"=w172) -> ("Dummy Test Handle Out"=w167:T43, "error out"=w171:errorcluster)  [unwired: 11 in, 1 out]
          n52 = call "niDTS BT EDR Tx Test Initiate.vi"("Dummy Test Handle In"=w167, "error in (no error)"=w171) -> ("Dummy Test Handle Out"=w166:T43, "error out"=w147:errorcluster)  [unwired: 12 in]
          n53 = call "niDTS BT EDR Tx Test Fetch Results.vi"("Dummy Test Handle in"=w166, "error in (no error)"=w147) -> ("Dummy Test Handle out"=w165:T43, "EDR Resutls"=w149:T17, "error out"=w170:errorcluster)  [unwired: 11 in]
          "EDR Results" <- w149
          n54 = Greater?(x=w149, y=w153) -> (0:→"EDR":T45)
          n55 = Less?(x=w149, y=w152) -> (x < y?=→"EDR":T45)
          n56 = call "niDTS BT EDR Tx Test Close.vi"("Dummy Test Handle out"=w165, "error in (no error)"=w170) -> ("error out"=w148:errorcluster)  [unwired: 13 in]
        }
      }
    }
    frame "LE TP" {
      n57 = flat-sequence {
        tunnel: w181 -> [w197]
        tunnel: [w198] -> w180
        tunnel: w179 -> [w196]
        tunnel: w178 -> [w195]
        tunnel: w177 -> [w211]
        tunnel: w176 -> [w194]
        tunnel: w175 -> [w193]
        frame #0 {
          # "BT LE Tx Test Step"
          n58 = call "niDTS BT LE Tx Test Initialize.vi"("Dut Reference"=w211, "SystemTechnologyCatalog"=w196, "SystemDut"=w195, "Logger Reference"=w194, "error in (no error)"=w197) -> ("Dummy Test Handle out"=w210:T43, "error out"=w209:errorcluster)  [unwired: 8 in, 1 out]
          n59 = call "niDTS BT LE Tx Test Get Default Parameters.vi"("Dummy Test Handle In"=w210, "error in (no error)"=w209) -> ("Dummy Test Handle Out"=w184:T43, "LE Tx Parameters"=w182:T30, "error out"=w183:errorcluster)  [unwired: 11 in]
          n60 = call "niDTS BT LE Tx Test Set Parameters.vi"("Dummy Test Handle In"=w184, "Parameters"=w182, "error in (no error)"=w183) -> ("Dummy Test Handle Out"=w208:T43, "error out"=w207:errorcluster)  [unwired: 11 in]
          n61 = call "niDTS BT LE Tx Test Configure.vi"("Dummy Test Handle In"=w208, "LE Tx Input Parameters"="LE Tx Input Parameters", "ResultsIndex"=w193, "error in (no error)"=w207) -> ("Dummy Test Handle Out"=w206:T43, "error out"=w205:errorcluster)  [unwired: 10 in]
          n62 = call "niDTS BT LE Tx Test Get Default Limits.vi"("Dummy Test Handle In"=w206, "error in (no error)"=w205) -> ("Dummy Test Handle Out"=w204:T43, "USL"=w188:T28, "LSL"=w187:T28, "error out"=w203:errorcluster)  [unwired: 10 in]
          "LE USL" <- w188
          "LE LSL" <- w187
          n63 = call "niDTS BT LE Tx Test Get Documentation.vi"("Dummy Test Handle In"=w204, "error in (no error)"=w203) -> ("Dummy Test Handle Out"=w202:T43, "error out"=w201:errorcluster)  [unwired: 11 in, 1 out]
          n64 = call "niDTS BT LE Tx Test Initiate.vi"("Dummy Test Handle In"=w202, "error in (no error)"=w201) -> ("Dummy Test Handle Out"=w200:T43, "error out"=w192:errorcluster)  [unwired: 12 in]
          n65 = call "niDTS BT LE Tx Test Fetch Results.vi"("Dummy Test Handle in"=w200, "error in (no error)"=w192) -> ("Dummy Test Handle out"=w185:T43, "Results"=w191:T28, "error out"=w199:errorcluster)  [unwired: 11 in]
          "LE Results" <- w191
          n66 = Greater?(x=w191, y=w187) -> (0:→"x > y?":T46)
          n67 = Less?(x=w191, y=w188) -> (x < y?=→"x < y?":T46)
          n68 = call "niDTS BT LE Tx Test Close.vi"("Dummy Test Handle out"=w185, "error in (no error)"=w199) -> ("error out"=w198:errorcluster)  [unwired: 13 in]
        }
      }
    }
  }
  n69 = flat-sequence {
    tunnel: w18 -> [w213]
    tunnel: w21 -> [w217]
    tunnel: w12 -> [w216]
    tunnel: w11 -> [w214]
    tunnel: [w212] -> w2
    tunnel: [w213] -> w1
    tunnel: [w222] -> w20
    tunnel: w2 -> [w224]
    tunnel: w1 -> [w227]
    frame #0 {
      # "TestStand Model Plugin Close"
      n70 = flat-sequence {
        tunnel: w217 -> [w220]
        tunnel: [w219] -> w215
        tunnel: w216 -> [w218]
        frame #0 {
          # "Dut Handles Cleanup"
          n71 = call "niDTS TestStand Station Close Dut Handles.vi"("Socket Dut Handles In"=w218, "Close All"=TRUE, "error in (no error)"=w220) -> ("error out"=w219:errorcluster)  [unwired: 11 in, 1 out]
        }
      }
      n72 = call "niDTS TestStand Station Close Instrument Catalog.vi"("Socket Instrument Catalog"=w214, "error in (no error)"=w215) -> ("error out"=w212:errorcluster)  [unwired: 13 in]
    }
    frame #1 {
      n73 = case shown="True" "Keep Log Open" {
        selector: "Keep Log Open" -> [w228 w230]
        tunnel: w224 -> [w229 w234]
        tunnel: [w229 w234] -> w223
        tunnel: [w228 w230] -> w226
        frame False {
        }
        frame True {
          n74 = property on="Keep Log Open" class="Bool (strict)"("Blinking"=w230) -> (error out=w231:errorcluster)  [unwired: 2 in, 1 out]
          n75 = while {
            tunnel: [w238] -> w232
            tunnel: w231 -> [w237]
            stop <- w236 stop-if-true
            n76 = property on="Keep Log Open" class="Bool (strict)"(error in=w237) -> (error out=w238:errorcluster, "Value"=w235:bool)  [unwired: 1 in, 1 out]
            n77 = Not(x=w235) -> (.not. x?=w236:bool)
            n78 = Wait (ms)(milliseconds to wait=u32 100) -> ()  [unwired: 1 out]
          }
          n79 = property on="Keep Log Open" class="Bool (strict)"(error in=w232, "Blinking"=FALSE) -> ()  [unwired: 1 in, 2 out]
        }
      }
      n80 = property on="Keep Log Open" class="Bool (strict)"("Value"=w226) -> ()  [unwired: 2 in, 2 out]
      n81 = call "niDTS Logger Close.vi"("Logger Handle in"=w227, "error in (no error)"=w223) -> ("error out"=w222:errorcluster)  [unwired: 13 in]
    }
  }
  "error out" <- w20
